vi "Mode Write.vi"(4 "error in (no error)":errorcluster, 5 "Value":T1, 6 "Container State":T4, 7 "Display State In":T2) -> (0 "error out":errorcluster, 3 "Display State Out":T2)   [LabVIEW 2013, in "UI_TimeSelector.xctl"]
uses:
  UI_TimeSelector.xctl
  <vilib>/_xctls/Container State.ctl
  State.ctl
  Typedefs/INTERNAL-DATA.ctl
  Interface/DEF-Mode.ctl
  <vilib>/_xctls/XControlSupport.lvlib
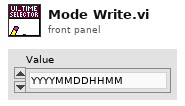
[diagram p1: front panel]
types:
  T1 = typedef "UI_TimeSelector.xctl/DEF-Mode.ctl" = enum16{"YYYYMMDDHHMM", "YYYYMMDDHHMMSS", "YYYY", "YYYYMM", "YYYYMMDD", "HHMM", "HHMMSS"}
  T2 = typedef "UI_TimeSelector.xctl/State.ctl" = cluster{"data":T3, "mode":T1}
  T3 = typedef "UI_TimeSelector.xctl/INTERNAL-DATA.ctl" = cluster{"year":string, "month":string, "day":string, "hour":string, "minute":string, "second":string}
  T4 = typedef "XControlSupport.lvlib/Container State.ctl" = cluster{"Indicator?":bool, "Run Mode?":bool, " Refnum":refnum<vi>}
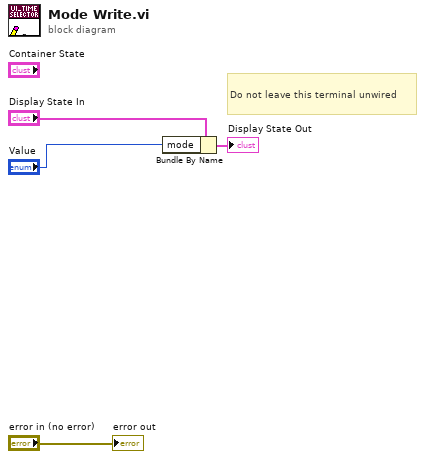
[diagram p0: block diagram]
diagram:
  # "Do not leave this terminal unwired"
  n1 = Bundle By Name(cluster="Display State In", "mode"="Value") -> (→"Display State Out":T2)
  "error out" <- "error in (no error)"
